vi "Create Orthogonal Polynomial.vi"(9 "alpha":dbl, 10 "order":i32, 11 "type":T1(ring)) -> (0 "error":i32, 3 "P(x)":dbl[](array[numeric]))   [LabVIEW 2020, in "NI_AALPro.lvlib"]
doc: "Creates orthogonal polynomial coefficients."
uses:
  NI_AALPro.lvlib
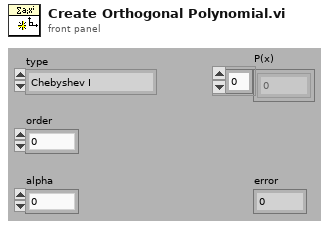
[diagram p1: front panel]
types:
  T1 = enum16{"Chebyshev I", "Chebyshev II", "Legendre", "Laguerre", "Hermite", "Associate Laguerre", "Gegenbauer"}
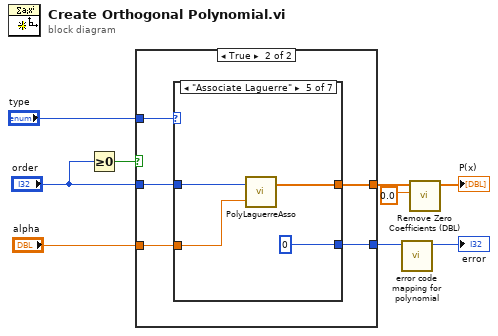
[diagram p0: block diagram]
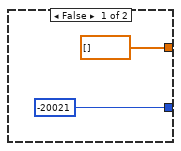
[diagram p2: hidden frame]
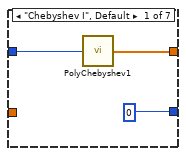
[diagram p3: hidden frame]
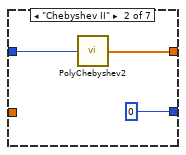
[diagram p4: hidden frame]
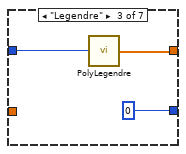
[diagram p5: hidden frame]
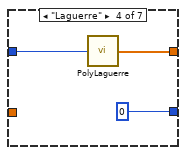
[diagram p6: hidden frame]
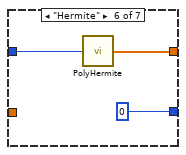
[diagram p7: hidden frame]
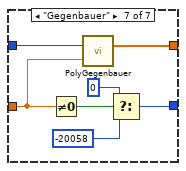
[diagram p8: hidden frame]
diagram:
  n1 = Greater Or Equal To 0?(x="order") -> (x >= 0?=w6:bool)
  n2 = case shown="True" w6 {
    tunnel: "type" -> [_ w16]
    tunnel: "order" -> [_ w15]
    tunnel: "alpha" -> [_ w14]
    tunnel: [dbl[] [] ("BDL") w13] -> w5
    tunnel: [-20021 ("minus order") w12] -> w2
    frame False {
    }
    frame True {
      n3 = case shown="\"Associate Laguerre\"" w16 {
        tunnel: w15 -> [w19 w22 w25 w28 w32 w35 w42]
        tunnel: w14 -> [_ _ _ _ w31 _ w40]
        tunnel: [w18 w21 w24 w27 w30 w34 w41] -> w13
        tunnel: [0 0 ("DimensionErr") 0 ("DimensionErr") 0 ("DimensionErr") 0 ("DimensionErr") 0 ("DimensionErr") w36] -> w12
        frame "Chebyshev I", Default {
          n4 = call "PolyChebyshev1.vi"("n"=w19) -> ("Tn"=w18:dbl[])
        }
        frame "Chebyshev II" {
          n5 = call "PolyChebyshev2.vi"("n"=w22) -> ("Un"=w21:dbl[])
        }
        frame "Legendre" {
          n6 = call "PolyLegendre.vi"("n"=w25) -> ("Pn"=w24:dbl[])
        }
        frame "Laguerre" {
          n7 = call "PolyLaguerre.vi"("n"=w28) -> ("Ln"=w27:dbl[])
        }
        frame "Associate Laguerre" {
          n8 = call "PolyLaguerreAsso.vi"("alpha"=w31, "n"=w32) -> ("Lna"=w30:dbl[])
        }
        frame "Hermite" {
          n9 = call "PolyHermite.vi"("n"=w35) -> ("Hn"=w34:dbl[])
        }
        frame "Gegenbauer" {
          n10 = Not Equal To 0?(x=w40) -> (x != 0?=w39:bool)
          n11 = call "PolyGegenbauer.vi"("alpha"=w40, "n"=w42) -> ("Cna"=w41:dbl[])
          n12 = Select(t=0, s=w39, f=-20058 ("DimensionErr")) -> (s? t:f=w36:i32)
        }
      }
    }
  }
  n13 = call "error code mapping for polynomial.vi"("error in"=w2) -> ("error out"=→"error":i32)  [unwired: 10 in]
  n14 = call "Remove Zero Coefficients (DBL).vi"("threshold"=0.0, "P(x) In"=w5) -> ("P(x) Out"=→"P(x)":dbl[])  [unwired: 7 in, 2 out]
